vi "Test ATM Deposit Updates Account Database.vi"(8 "error in (no error)":errorcluster, 11 "Test Case In":refnum<class "Controller Test.lvclass">) -> (0 "error out":errorcluster, 3 "Test Case Out":refnum<class "Controller Test.lvclass">)   [LabVIEW 2020, in "Controller Test.lvclass"]
uses:
  Controller Test/Controller Test.lvclass
  C:/Program Files (x86)/National Instruments/LabVIEW 2020/vi.lib/Astemes/LUnit/Test Case.lvclass
  Account Database/Account Data.ctl
  <vilib>/Astemes/LUnit/Test Case.lvclass/Test Case.ctl
  01074fa8-ee8a-411d-bc8b-fc92c4f90959.vi
  <vilib>/Astemes/LUnit/Palette/Pass.vi
  <vilib>/Astemes/LUnit/Palette/Fail.vi
  <vilib>/Astemes/LUnit/Compare Variants.vi
  <vilib>/Astemes/LUnit/Describe Comparison.vi
  <vilib>/Astemes/LUnit/Set Assertion Type.vi
  <vilib>/Astemes/LUnit/Add test result.vi
  <vilib>/Astemes/LUnit/Variant to string.vi
  <vilib>/Astemes/LUnit/LUnit Record Assertion Result.vi
  <vilib>/Astemes/LUnit/LUnit Aggregate Assertion Results.vi
  <vilib>/Astemes/LUnit/Method Result/LUnit Merge Status.vi
  <vilib>/Astemes/LUnit/LUnit Concatenate result strings.vi
  <vilib>/Utility/Data Type/Get Type Information.vi
  <vilib>/Utility/LVClass/Get LV Class Name.vi
  Controller Test/Controller Test.lvclass/Controller Test.ctl
  ATM Controller/ATM Controller.lvclass
  Account Database/Account Database.lvclass
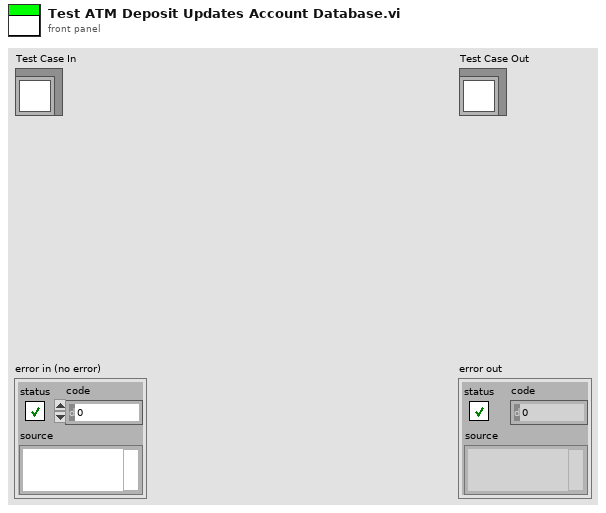
[diagram p1: front panel]
types:
  T1 = typedef "Account Database.lvclass/Account Data.ctl" = cluster{"Account Number":string, "First Name":string, "Last Name":string, "Account Balance":string}
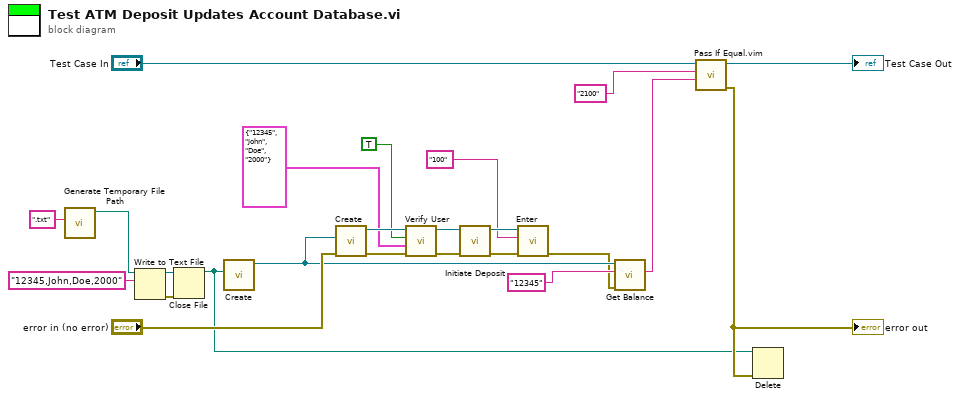
[diagram p0: block diagram]
diagram:
  n1 = call <vilib>:"Generate Temporary File Path.vi"("Temporary File Extension (tmp)"=".txt") -> ("Unique Temporary File Path"=w10:path)  [unwired: 9 in, 1 out]
  n2 = Write to Text File(file (use dialog)=w10, text="12345,John,Doe,2000") -> (refnum out=w8:refnum<file>, error out=w9:errorcluster)  [unwired: 2 in, 1 out]
  n3 = Close File(refnum=w8, error in=w9) -> (path=w1:path)  [unwired: 1 out]
  n4 = call "Create.vi"("Data File"=w1) -> ("Account Database out"=w7:refnum<class "Account Database.lvclass">)  [unwired: 9 in, 1 out]
  n5 = call "Create.vi"("error in (no error)"="error in (no error)", "Account Database"=w7) -> ("error out"=w21:errorcluster, "ATM Controller out"=w16:refnum<class "ATM Controller.lvclass">)  [unwired: 8 in]
  n6 = call "Verify User.vi"("error in (no error)"=w21, "Account Data"=T1 {"Account Number"="12345", "First Name"="John", "Last Name"="Doe", "Account Balance"="2000"}, "Verified?"=TRUE, "ATM Controller in"=w16) -> ("error out"=w17:errorcluster, "ATM Controller out"=w15:refnum<class "ATM Controller.lvclass">)  [unwired: 6 in]
  n7 = call "Initiate Deposit.vi"("error in (no error)"=w17, "ATM Controller in"=w15) -> ("error out"=w19:errorcluster, "ATM Controller out"=w20:refnum<class "ATM Controller.lvclass">)  [unwired: 8 in]
  n8 = call "Enter.vi"("error in (no error)"=w19, "User Input"="100", "ATM Controller in"=w20) -> ("error out"=w5:errorcluster)  [unwired: 7 in, 1 out]
  n9 = call "Get Balance.vi"("error in (no error)"=w5, "Account Number"="12345", "Account Database in"=w7) -> ("Account Balance"=w4:string)  [unwired: 6 in, 2 out]
  n10 = call "Pass If Equal.vim"("Actual"=w4, "Expected"="2100" ("Account Balance"), "LUnit Test Case In"="Test Case In") -> ("error out"=w2:errorcluster, "LUnit Test Case Out"=→"Test Case Out":refnum<class "Controller Test.lvclass">)  [unwired: 7 in]
  "error out" <- w2
  n11 = Delete(path (use dialog)=w1, error in=w2) -> ()  [unwired: 3 in, 3 out]
